vi "Vision Research Phantom Series PhCon PhGetCineParams.vi"(0 "CN in":u32=1, 1 "Cine":T1 items=["CINE_DEFAULT "=-2, "CINE_CURRENT "=-1, "CINE_PREVIEW  "=0, "CINE_FIRST    "=1, "FIRST_FLASH_CINE"=101], 5 "Error In (no error)":errorcluster) -> (14 "CN out":u32=1, 15 "Cine out":T1 items=["CINE_DEFAULT "=-2, "CINE_CURRENT "=-1, "CINE_PREVIEW  "=0, "CINE_FIRST    "=1, "FIRST_FLASH_CINE"=101], 16 "ACQUIPARAMS":T2 {"CFA"."CFA" items=["CFA_NONE", "CFA_VRI", "CFA_VRIV6", "CFA_BAYER", "CFA_BAYERFLIP"]; "TriggerTime"."fractions" format="%32.0f"}, 17 "pBMI":T7, 19 "Error Out":errorcluster)   [LabVIEW 2013, in "VRI.lvlib"]
doc: "PhCon.dll\n\nPhGetCineParams\nHRESULT PhGetCineParams(UINT CN, INT Cine, PACQUIPARAMS pParams, PBITMAPINFO pBMI);\n\nParameters Description\nCN (in) Camera number.\nCine (in) Cine number\npAcquiParams (out) Pointer to the ACQUIPARAMS used when the cine was recorded.\npBMI (out) Pointer to the bitmapinfo of the image filled by this routine.\nReturn HRESULT (0=Ok)\nComments Read the parameters used to record the cine from the camera \n memory and fill an image header. Please allocate space for \n the BITMAPINFOHEADER and for the the gray palette \n (256*sizeof(RGBQUAD) ). Both parameters may be NULL.\n\nWritten by:\nBLOOMY CONTROLS, INC\nWINDSOR, CT 06095, USA\n860-298-9925\nwww.bloomy.com\nV1.0.0\nMay, 2004"
uses:
  VRI.lvlib
  _Type Defs/PhCon Predefined Cines.ctl
  _Type Defs/BITMAPINFO.ctl
  _Type Defs/BITMAPINFOHEADER.ctl
  _Type Defs/RGBQUAD.ctl
  _Type Defs/PHCon ACQUIPARAMS.ctl
  _Type Defs/PhCon SyncImaging.ctl
  _Type Defs/Rect.ctl
  _Type Defs/PHCon Time64.ctl
  _Type Defs/PhInt CFA.ctl
  Phantom DLLs/PhCon.dll
panel:
  out "pBMI Data":u8[](array[numeric])
  out "pParams Data":u32[](array[numeric])
  # "For instructions on the use of this VI, press Ctrl+H to display the help window and move the mouse over the icon, controls, and indicators"
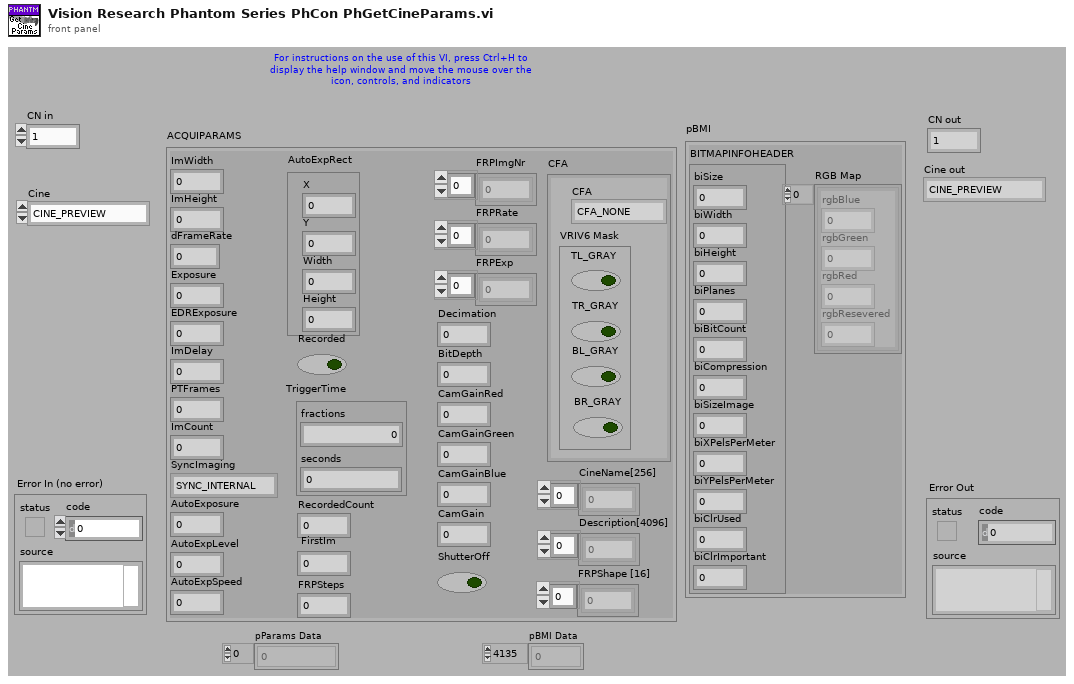
[diagram p1: front panel]
types:
  T1 = typedef "VRI.lvlib/PhCon Predefined Cines.ctl" = i32
  T2 = typedef "VRI.lvlib/PHCon ACQUIPARAMS.ctl" = cluster{"ImWidth":u32, "ImHeight":u32, "(deprecated)FrameRateInt":u32, "Exposure":u32, "EDRExposure":u32, "ImDelay":u32, "PTFrames":u32, "ImCount":u32, "SyncImaging":T3, "AutoExposure":u32, "AutoExpLevel":u32, "AutoExpSpeed":u32, "AutoExpRect":T4, "Recorded":bool, "TriggerTime":T5, "RecordedCount":u32, "FirstIm":i32, "FRPSteps":u32, "FRPImgNr":i32[], "FRPRate":u32[], "FRPExp":u32[], "Decimation":u32, "BitDepth":u32, "CamGainRed":u32, "CamGainGreen":u32, "CamGainBlue":u32, "CamGain":u32, "ShutterOff":bool, "CFA":T6, "CineName[256]":u8[], "Description[4096]":u8[], "FRPShape [16]":u32[], "dFrameRate":dbl}
  T3 = typedef "VRI.lvlib/PhCon SyncImaging.ctl" = enum32{"SYNC_INTERNAL", "SYNC_EXTERNAL", "SYNC_LOCKTOIRIG"}
  T4 = typedef "VRI.lvlib/Rect.ctl" = cluster{"X":i32, "Y":i32, "Width":i32, "Height":i32}
  T5 = typedef "VRI.lvlib/PHCon Time64.ctl" = cluster{"fractions":u32, "seconds":u32}
  T6 = typedef "VRI.lvlib/PhInt CFA.ctl" = cluster{"CFA":u32, "VRIV6 Mask":cluster{"TL_GRAY":bool, "TR_GRAY":bool, "BL_GRAY":bool, "BR_GRAY":bool}}
  T7 = typedef "VRI.lvlib/BITMAPINFO.ctl" = cluster{"BITMAPINFOHEADER":T8, "RGB Map":T9[]}
  T8 = typedef "VRI.lvlib/BITMAPINFOHEADER.ctl" = cluster{"biSize":u32, "biWidth":i32, "biHeight":i32, "biPlanes":u16, "biBitCount":u16, "biCompression":u32, "biSizeImage":u32, "biXPelsPerMeter":i32, "biYPelsPerMeter":i32, "biClrUsed":u32, "biClrImportant":u32}
  T9 = typedef "VRI.lvlib/RGBQUAD.ctl" = cluster{"rgbBlue":u8, "rgbGreen":u8, "rgbRed":u8, "rgbResevered":u8}
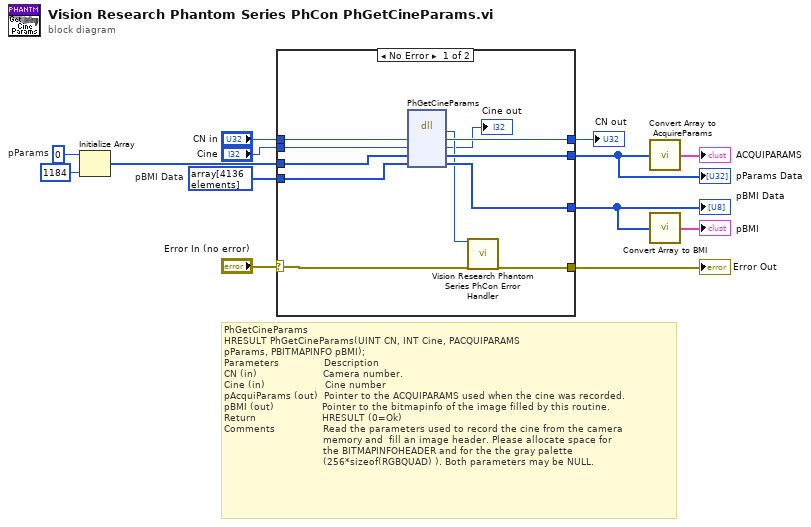
[diagram p0: block diagram]
diagram:
  w2 = u32 0  # pParams
  w8 = u8[] array[4136 elements]  # pBMI Data
  # "PhGetCineParams\nHRESULT PhGetCineParams(UINT CN, INT Cine, PACQUIPARAMS\npParams, PBITMAPINFO pBMI);\nParameters               Description\nCN (in)                      Camera number.\nCine (in)                    Cine number\npAcquiParams (out)  Pointer to the ACQUIPARAMS used when the cine was recorded.\npBMI (out)                Pointer to the bitmapinfo of the image filled by this routine.\nReturn                      HRESULT (0=Ok)\nComments                Read the parameters used to record the cine from the camera \n                                 memory and  fill an image header. Please allocate space for \n                                 the BITMAPINFOHEADER and for the the gray palette \n                                 (256*sizeof(RGBQUAD) ). Both parameters may be NULL."
  n1 = Initialize Array(w2, 1184 ("dimension size")) -> (w1:u32[])
  n2 = case shown="No Error" "Error In (no error)" {
    selector: "Error In (no error)" -> [w24 w28]
    tunnel: [w23 w28] -> w12
    tunnel: "CN in" -> [w22 w27]
    tunnel: [w21 w27] -> w10
    tunnel: "Cine" -> [w20 _]
    tunnel: w1 -> [w19 w26]
    tunnel: [w18 w26] -> w5
    tunnel: w8 -> [w17 w25]
    tunnel: [w16 w25] -> w4
    frame No Error {
      n3 = dll-call lib="C:/Projects/SDK/32-bit/Vision Research Phantom Series Labview Driver/Phantom DLLs/PhCon.dll" fn="PhGetCineParams"("CN"=w22, "Cine"=w20, "pParams"=w19, "pBMI"=w17) -> ("HRESULT"=w15:i32, "CN"=w21:u32, "Cine"=→"Cine out":i32, "pParams"=w18:u32[], "pBMI"=w16:u8[])  [unwired: 3 in, 2 out]
      n4 = call "Vision Research Phantom Series PhCon Error Handler.vi"("ErrNo"=w15, "Error In (no error)"=w24) -> ("Error Out"=w23:errorcluster)  [unwired: 17 out]
    }
    frame Error {
    }
  }
  "Error Out" <- w12
  "CN out" <- w10
  "pParams Data" <- w5
  "pBMI Data" <- w4
  n5 = call "Convert Array to AcquireParams.vi"("ACQUIPARAMS BYTE ARRAY"=w5) -> ("ACQUIPARAMS"=→"ACQUIPARAMS":T2)
  n6 = call "Convert Array to BMI.vi"("pBMI Data"=w4) -> ("pBMI"=→"pBMI":T7)
